vi "Get Ellipse Points.vi"(11 "Ellipse":T1) -> (3 "Points":cluster{dbl, dbl}[](array[cluster]))   [LabVIEW 2015, in "Digital Image Processing.lvlib"]
uses:
  Digital Image Processing.lvlib
  <vilib>/Analysis/1siggen.llb/Ramp Pattern by Samples.vi
  <vilib>/Analysis/NI_AALBase.lvlib
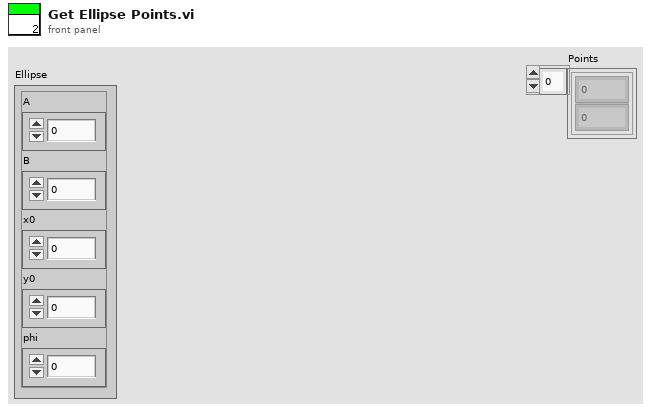
[diagram p1: front panel]
types:
  T1 = cluster{"A":dbl, "B":dbl, "x0":dbl, "y0":dbl, "phi":dbl}
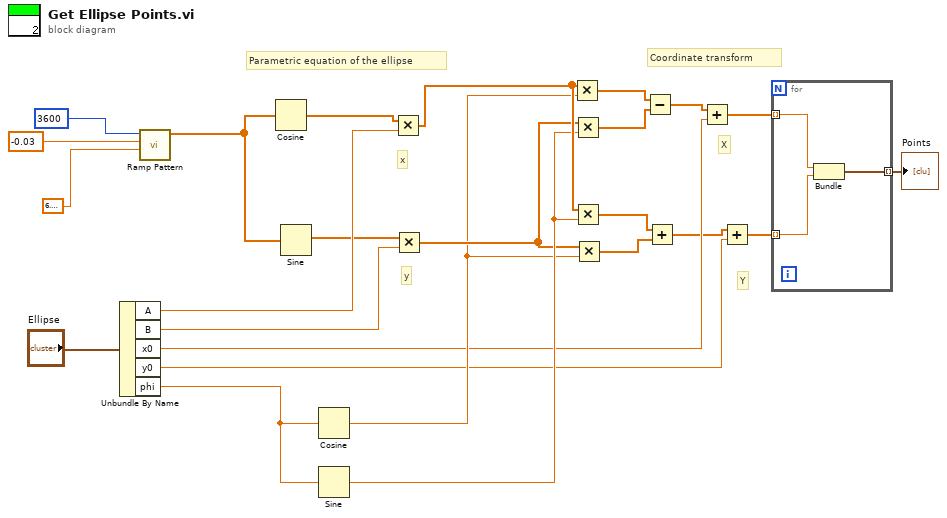
[diagram p0: block diagram]
diagram:
  # "Y"
  # "X"
  # "y"
  # "x"
  # "Coordinate transform"
  # "Parametric equation of the ellipse"
  n1 = Unbundle By Name("Ellipse") -> ("A"=w19:dbl, "B"=w17:dbl, "x0"=w6:dbl, "y0"=w4:dbl, "phi"=w16:dbl)
  n2 = call-poly <vilib>:"Ramp Pattern.vi"("start"=6.283185307179586, "end"=-0.03, "samples"=3600) -> ("Ramp Pattern"=w21:dbl[])  [unwired: 7 in, 1 out]
  n3 = Cosine(x=w21) -> (cos(x)=w20:dbl[])
  n4 = Sine(x=w21) -> (sin(x)=w18:dbl[])
  n5 = Cosine(x=w16) -> (cos(x)=w12:dbl)
  n6 = Sine(x=w16) -> (sin(x)=w14:dbl)
  n7 = Multiply(x=w20, y=w19) -> (x*y=w15:dbl[])
  n8 = Multiply(x=w18, y=w17) -> (x*y=w13:dbl[])
  n9 = Multiply(x=w15, y=w12) -> (x*y=w11:dbl[])
  n10 = Multiply(x=w13, y=w14) -> (x*y=w10:dbl[])
  n11 = Multiply(x=w15, y=w14) -> (x*y=w9:dbl[])
  n12 = Multiply(x=w13, y=w12) -> (x*y=w8:dbl[])
  n13 = Subtract(x=w11, y=w10) -> (x-y=w7:dbl[])
  n14 = Add(x=w9, y=w8) -> (x+y=w5:dbl[])
  n15 = Add(x=w7, y=w6) -> (x+y=w3:dbl[])
  n16 = Add(x=w5, y=w4) -> (x+y=w2:dbl[])
  n17 = for {
    tunnel: w3 -> [w28] mode=indexing
    tunnel: w2 -> [w27] mode=indexing
    tunnel: [w26] -> w1 mode=indexing
    n18 = Bundle(w28, w27) -> (w26:cluster{dbl, dbl})  [unwired: 1 in]
  }
  "Points" <- w1
